vi "Get Pane At Point.vi"(9 "Y":i32, 10 "X":i32, 11 "All Pane Details":T1[](array[typedef])) -> (2 "Found?":bool, 3 "Pane Index":i32)   [LabVIEW 2018]
uses:
  Typedefs/Pane Details--Cluster.ctl
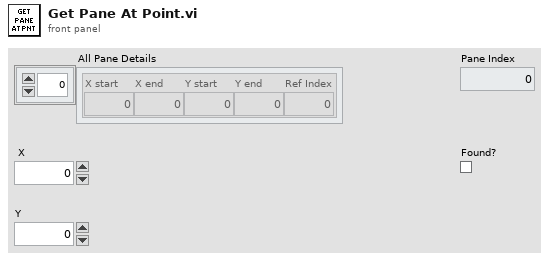
[diagram p1: front panel]
types:
  T1 = typedef "Pane Details--Cluster.ctl" = cluster{"X start":i32, "X end":i32, "Y start":i32, "Y end":i32, "Ref Index":i32}
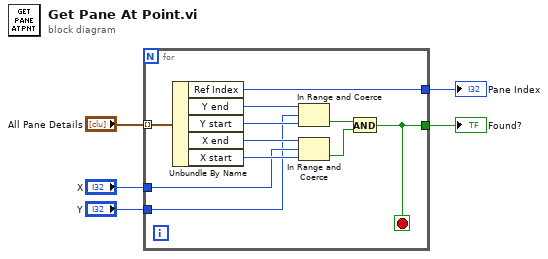
[diagram p0: block diagram]
diagram:
  n1 = for {
    tunnel: "All Pane Details" -> [w16] mode=indexing
    tunnel: "X" -> [w9]
    tunnel: "Y" -> [w8]
    tunnel: [w7] -> w5
    tunnel: [w6] -> w1
    stop <- w7 stop-if-true
    n2 = Unbundle By Name(w16) -> ("Ref Index"=w6:i32, "Y end"=w15:i32, "Y start"=w14:i32, "X end"=w13:i32, "X start"=w12:i32)
    n3 = In Range and Coerce(upper limit=w15, x=w8, lower limit=w14) -> (In Range?=w11:bool)  [unwired: 1 out]
    n4 = In Range and Coerce(upper limit=w13, x=w9, lower limit=w12) -> (In Range?=w10:bool)  [unwired: 1 out]
    n5 = And(x=w11, y=w10) -> (x .and. y?=w7:bool)
  }
  "Found?" <- w5
  "Pane Index" <- w1
